vi "Config Select Dialog.vi"(8 "Error In":errorcluster, 11 "Message Queue":refnum<queue>) -> (0 "Error Out":errorcluster, 2 "Msg out":string)   [LabVIEW 2014]
uses:
  APIs/Message Queue/Message Cluster.ctl
  APIs/Message Queue/Enqueue Message (Single).vi
  APIs/Message Queue/WINFAS 2 Message Queue.lvlib
panel:
  in  "Selector HWAsync":T1
  in  "Selector HWSync":T2
  # "HW Síncrono"
  # "HW Asíncrono"
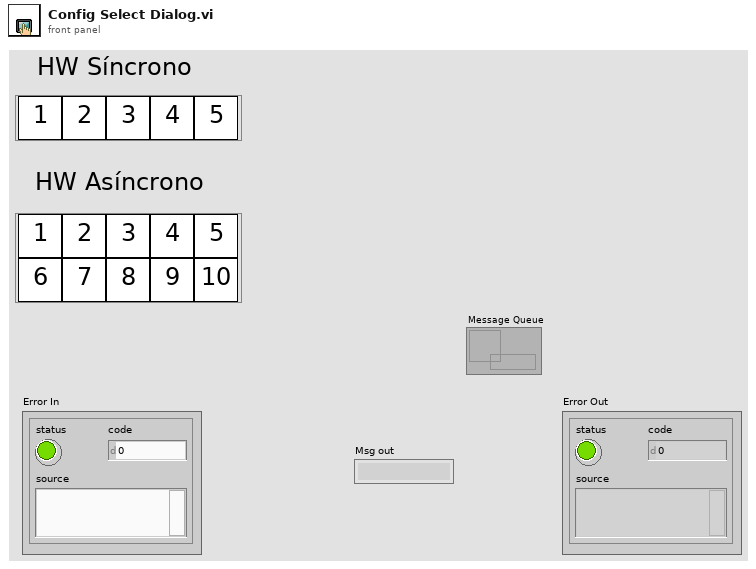
[diagram p1: front panel]
types:
  T1 = cluster{"Config 1":bool, "Config 2":bool, "Config 3":bool, "Config 4":bool, "Config 5":bool, "Config 6":bool, "Config 7":bool, "Config 8":bool, "Config 9":bool, "Config 10":bool}
  T2 = cluster{"Config 1":bool, "Config 2":bool, "Config 3":bool, "Config 4":bool, "Config 5":bool}
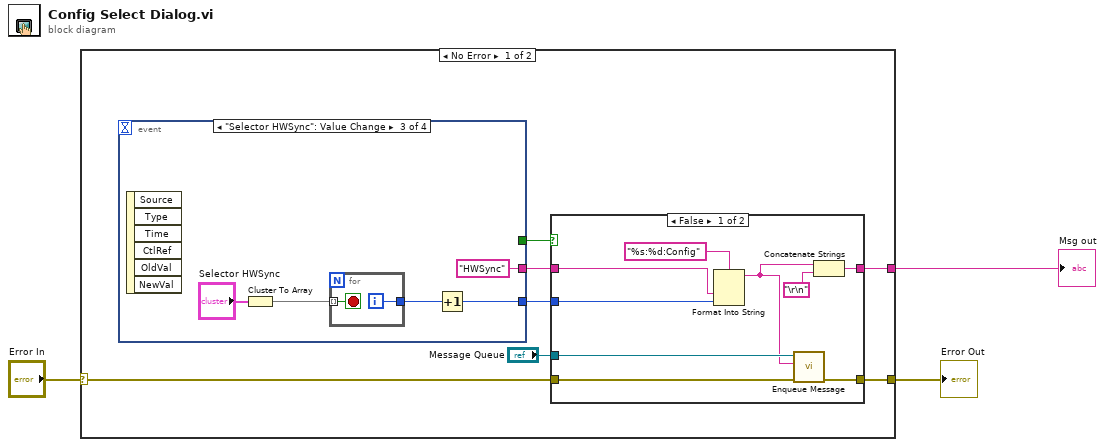
[diagram p0: block diagram]
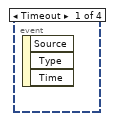
[diagram p3: hidden frame]
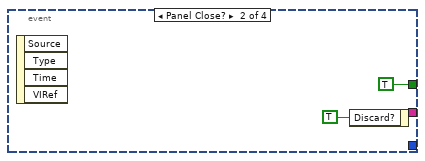
[diagram p4: hidden frame]
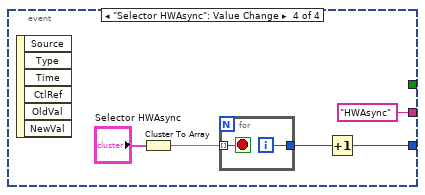
[diagram p5: hidden frame]
diagram:
  n1 = case shown="No Error" "Error In" {
    selector: "Error In" -> [w9 w37]
    tunnel: [w6 _] -> w3
    tunnel: [w8 w37] -> w1
    frame No Error {
      n2 = event shown="[2] \"Selector HWSync\": Value Change" {
        selector: _ -> [_ _ _ _]
        dyn-events: _ -> [_ _ _ _]
        timeout: _ -> [_ _ _ _]
        tunnel: [_ TRUE ("Discard?") _ _] -> w7
        tunnel: [_ _ w26 w34] -> w5
        tunnel: [_ _ "HWSync" ("format string") "HWAsync" ("format string")] -> w4
        event Timeout {
          n3 = event-data() -> ()  [unwired: 1 in, 3 out]
        }
        event Panel Close? {
          n4 = event-data() -> ()  [unwired: 1 in, 4 out]
          n5 = event-data("Discard?"=TRUE) -> ()  [unwired: 1 in, 1 out]
        }
        event "Selector HWSync": Value Change {
          n6 = event-data() -> ()  [unwired: 1 in, 6 out]
          n7 = Cluster To Array(cluster="Selector HWSync") -> (array=w24:bool[])
          n8 = for {
            tunnel: w24 -> [w28] mode=indexing
            tunnel: [w29] -> w23
            i -> [w29]
            stop <- w28 stop-if-true
          }
          n9 = Increment(x=w23) -> (x+1=w26:i32)
        }
        event "Selector HWAsync": Value Change {
          n10 = event-data() -> ()  [unwired: 1 in, 6 out]
          n11 = Cluster To Array(cluster="Selector HWAsync") -> (array=w31:bool[])
          n12 = for {
            tunnel: w31 -> [w35] mode=indexing
            tunnel: [w36] -> w30
            i -> [w36]
            stop <- w35 stop-if-true
          }
          n13 = Increment(x=w30) -> (x+1=w34:i32)
        }
      }
      n14 = case shown="False" w7 {
        tunnel: "Message Queue" -> [w19 _]
        tunnel: w9 -> [w18 w20]
        tunnel: [w17 w20] -> w8
        tunnel: [w15 _] -> w6
        tunnel: w5 -> [w12 _]
        tunnel: w4 -> [w11 _]
        frame False {
          n15 = Format Into String(format string="%s:%d:Config", w11, w12) -> (resulting string=w13:string)  [unwired: 2 in, 1 out]
          n16 = call-poly "Enqueue Message.vi"("error in (no error)"=w18, "Message"=w13, "Message Queue"=w19) -> ("error out"=w17:errorcluster)  [unwired: 7 in, 1 out]
          n17 = Concatenate Strings(w13, "\r\n") -> (w15:string)
        }
        frame True {
        }
      }
    }
    frame Error {
    }
  }
  "Msg out" <- w3
  "Error Out" <- w1
